vi "kADPosMerge.vi"(8 "Mismatch Tol":dbl=0.1, 9 "EncoderCountTimed":i32, 10 "B Analog Encoder Sync":i16, 11 "A Analog Encoder Sync":i16) -> (1 "AD Mismatch":u16, 3 "Final Position":dbl)   [LabVIEW 2010, in "KevLib01.lvlib"]
uses:
  KevLib01.lvlib
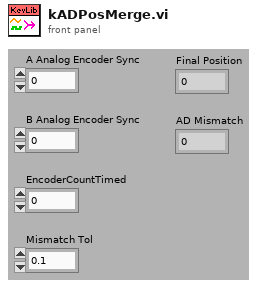
[diagram p1: front panel]
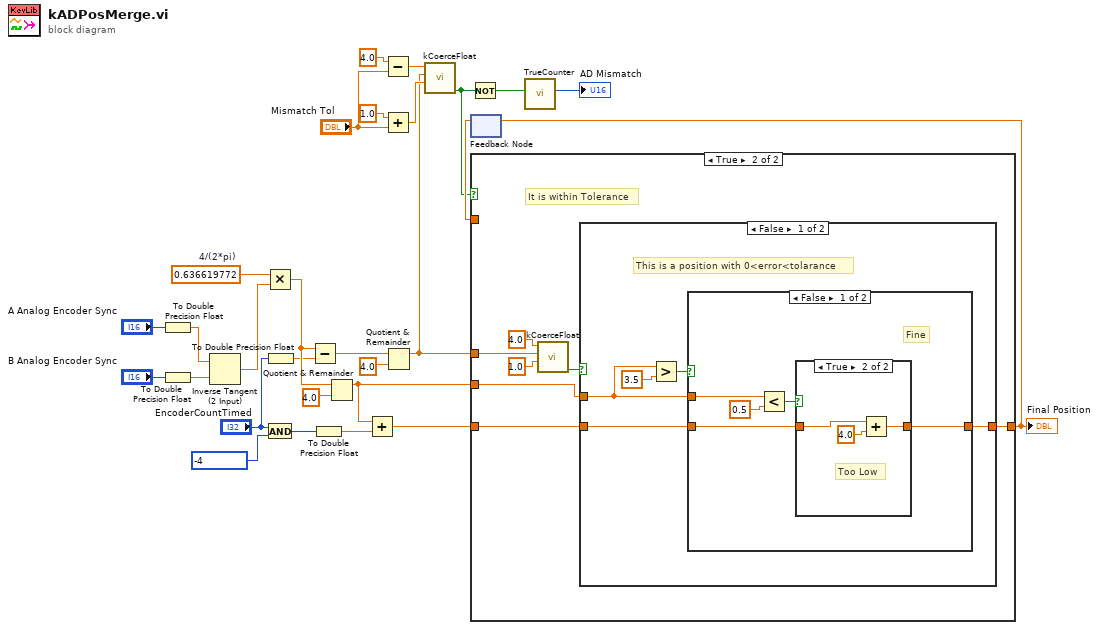
[diagram p0: block diagram]
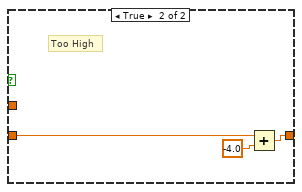
[diagram p4: hidden frame]
diagram:
  w18 = 0.636619772  # 4/(2*pi)
  n1 = To Double Precision Float(number="A Analog Encoder Sync") -> (double precision float=w7:dbl)
  n2 = To Double Precision Float(number="B Analog Encoder Sync") -> (double precision float=w8:dbl)
  n3 = Inverse Tangent (2 Input)(1:w8, 2:w7) -> (0:w17:dbl)
  n4 = Multiply(x=w18, y=w17) -> (x*y=w20:dbl)
  n5 = And(x="EncoderCountTimed", y=-4) -> (x .and. y?=w22:i32)
  n6 = To Double Precision Float(number="EncoderCountTimed") -> (double precision float=w16:dbl)
  n7 = Subtract(x=w20, y=w16) -> (x-y=w11:dbl)
  n8 = To Double Precision Float(number=w22) -> (double precision float=w23:dbl)
  n9 = Quotient & Remainder(x=w20, y=4.0) -> (x-y*floor(x/y)=w28:dbl)  [unwired: 1 out]
  n10 = Add(x=w28, y=w23) -> (x+y=w27:dbl)
  n11 = Subtract(x=4.0 ("y"), y="Mismatch Tol") -> (x-y=w5:dbl)
  n12 = Add(x=1.0 ("y"), y="Mismatch Tol") -> (x+y=w4:dbl)
  n13 = Quotient & Remainder(x=w11, y=4.0) -> (x-y*floor(x/y)=w3:dbl)  [unwired: 1 out]
  n14 = call "kCoerceFloat.vi"("lower"=w4, "input"=w3, "upper"=w5) -> ("coerced?"=w2:bool)  [unwired: 8 out]
  n15 = Not(x=w2) -> (.not. x?=w1:bool)
  n16 = feedback #1() -> (w24:dbl)  [unwired: 1 out]
  n17 = case shown="True" w2 {
    tunnel: w24 -> [w29 _]
    tunnel: [w29 w36] -> w25
    tunnel: w27 -> [_ w35]
    tunnel: w3 -> [_ w31]
    tunnel: w28 -> [_ w34]
    frame False {
    }
    frame True {
      # "It is within Tolerance"
      n18 = call "kCoerceFloat.vi"("lower"=1.0 ("y"), "input"=w31, "upper"=4.0 ("y")) -> ("coerced?"=w30:bool)  [unwired: 8 out]
      n19 = case shown="False" w30 {
        tunnel: [w39 w54] -> w36
        tunnel: w35 -> [w38 w54]
        tunnel: w34 -> [w37 _]
        frame False {
          # "This is a position with 0<error<tolarance"
          n20 = Greater?(x=w37, y=3.5) -> (0:w41:bool)
          n21 = case shown="False" w41 {
            tunnel: [w43 w51] -> w39
            tunnel: w38 -> [w42 w53]
            tunnel: w37 -> [w45 _]
            frame False {
              # "Fine"
              n22 = Less?(x=w45, y=0.5) -> (x < y?=w44:bool)
              n23 = case shown="True" w44 {
                tunnel: [w47 w49] -> w43
                tunnel: w42 -> [w47 w50]
                frame False {
                  # "Fine"
                }
                frame True {
                  # "Too Low"
                  n24 = Add(x=w50, y=4.0) -> (x+y=w49:dbl)
                }
              }
            }
            frame True {
              # "Too High"
              n25 = Add(x=w53, y=-4.0) -> (x+y=w51:dbl)
            }
          }
        }
        frame True {
          # "Within Tolerance of 0"
        }
      }
    }
  }
  "Final Position" <- w25
  n26 = feedback-in #1(w25) -> ()
  n27 = call "TrueCounter.vi"("True?"=w1) -> ("True Count"=→"AD Mismatch":u16)  [unwired: 10 out]
